vi "isStaged.set.vi"(8 "error in":errorcluster, 10 "isStaged":bool, 11 "asset in":refnum<class "asset.lvclass">) -> (0 "error out":errorcluster, 3 "asset out":refnum<class "asset.lvclass">)   [LabVIEW 2020, in "asset.lvclass"]
uses:
  asset.lvclass
  asset.lvclass/asset.ctl
  Nominal Client/Nominal Client.lvclass
  6c9b2cde-d50a-4bef-9898-252f3db91ea5.vi
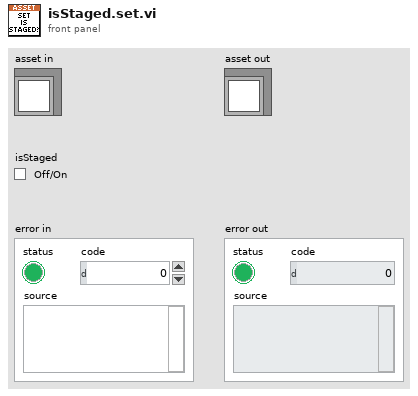
[diagram p1: front panel]
types:
  T1 = typedef "dataScopes.lvlib/links.ctl" = cluster{"URL":string, "Title":string}[]
  T2 = typedef "dataScopes.lvlib/data_scopes.ctl" = T3[]
  T3 = typedef "dataScopes.lvlib/data_scope.ctl" = cluster{"dataScopeName":string, "dataSource":T4, "seriesTags":refnum<class "properties.lvclass">, "offset":T6}
  T4 = typedef "dataScopes.lvlib/data_source.ctl" = cluster{"type":T5, "rid":string}
  T5 = typedef "dataScopes.lvlib/type.ctl" = enum16{"dataset", "connection", "logSet", "video"}
  T6 = typedef "dataScopes.lvlib/offset.ctl" = cluster{"seconds":i32, "nanos":i32, "picos":i32}
  T7 = cluster{"rid":string, "title":string, "properties":refnum<class "properties.lvclass">, "labels":refnum<class "labels.lvclass">, "Links":T1, "datascopes":T2, "createdAt":timestamp, "updatedAt":timestamp, "attachments":refnum<class "labels.lvclass">, "isStaged":bool, "isArchived":bool, "description":string, "createdBy":string, "type":string}
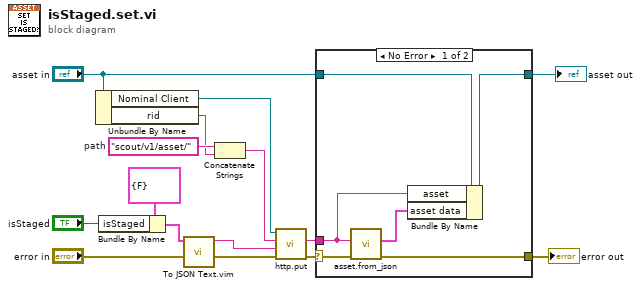
[diagram p0: block diagram]
diagram:
  w14 = "scout/v1/asset/"  # path
  n1 = Unbundle By Name("asset in") -> ("Nominal Client"=w15:refnum<class "Nominal Client.lvclass">, "rid"=w12:string)
  n2 = Bundle By Name(cluster=cluster{"isStaged":bool} {"isStaged"=FALSE}, "isStaged"="isStaged") -> (w2:cluster{"isStaged":bool})
  n3 = call "To JSON Text.vim"("error in (no error)"="error in", "Anything"=w2) -> ("error out"=w4:errorcluster, "<JSON>"=w5:string)  [unwired: 8 in]
  n4 = Concatenate Strings(w14, w12) -> (w13:string)
  n5 = call "http.put.vi"("error in"=w4, "Body"=w5, "Path"=w13, "Nominal Client in"=w15) -> ("error out"=w11:errorcluster, "Response"=w8:string)  [unwired: 4 in, 2 out]
  n6 = case shown="No Error" w11 {
    selector: w11 -> [w21 w23]
    tunnel: [w20 w23] -> w10
    tunnel: "asset in" -> [w19 w22]
    tunnel: w8 -> [w17 _]
    tunnel: [w16 w22] -> w7
    frame No Error {
      n7 = call "asset.from_json.vi"("error in"=w21, "asset"=w17) -> ("error out"=w20:errorcluster, "Asset Data"=w18:T7)  [unwired: 8 in]
      n8 = Bundle By Name(cluster=w19, "asset"=w17, "asset data"=w18) -> (w16:refnum<class "asset.lvclass">)
    }
    frame Error {
    }
  }
  "asset out" <- w7
  "error out" <- w10
